vi "ST5520_CMD.vi"(8 "errin":errorcluster caption="entrée d'erreur (pas d'erreur)", 10 "VISA":string) -> (0 "errout":errorcluster caption="sortie d'erreur", 1 "DATA FINAL FLT":dbl, 2 "DATA OUT":string, 3 "60s?":bool)   [LabVIEW 2020]
uses:
  OP500/VG/VG_progressBar.vi
panel:
  in  "Arrêter":bool
  out "DATA LIVE":string
  # "DATA OUT"
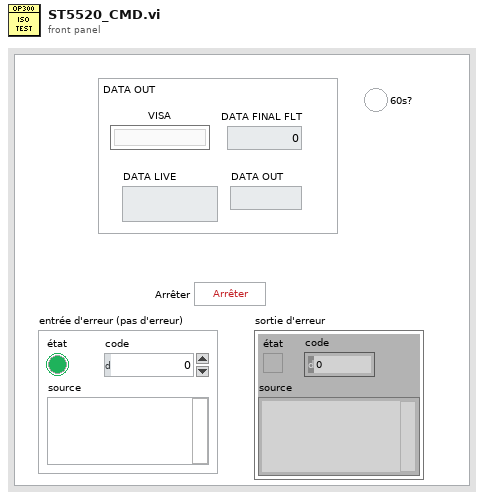
[diagram p1: front panel]
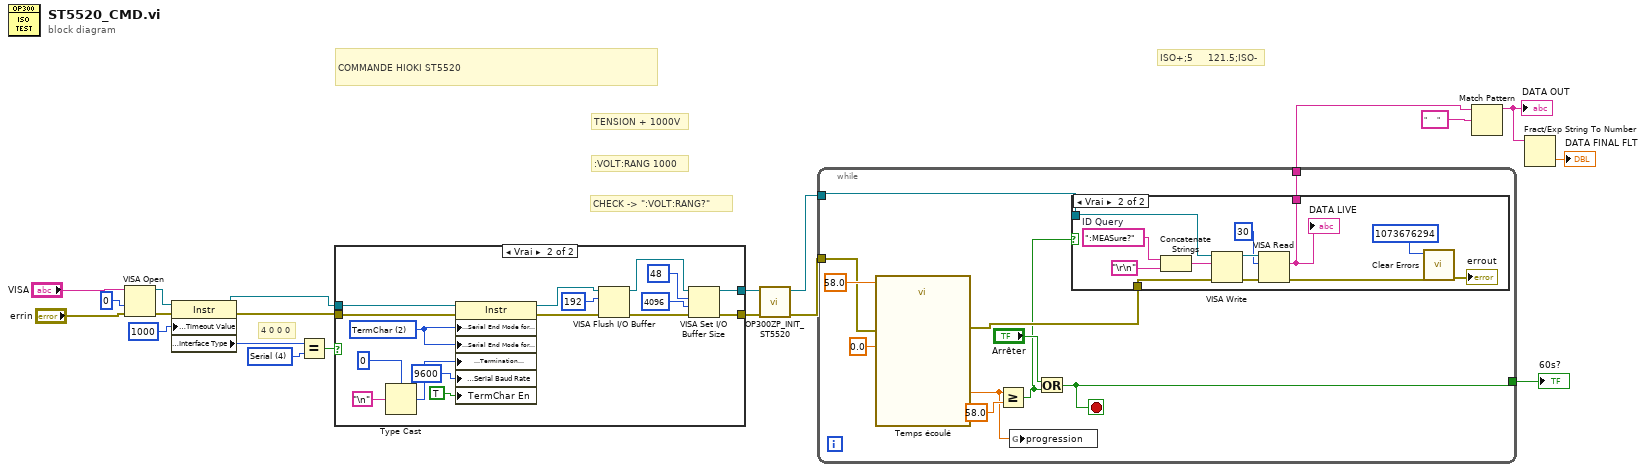
[diagram p0: block diagram]
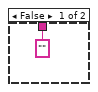
[diagram p3: hidden frame]
diagram:
  w11 = u16 4 items=["GPIB"=1, "VXI"=2, "GPIB-VXI"=3, "Serial"=4, "PXI"=5, "TCPIP"=6, "USB"=7] ("Interface Information:Interface Type")
  # "ISO+;5     121.5;ISO-"
  # "CHECK -> \":VOLT:RANG?\""
  # ":VOLT:RANG 1000"
  # "TENSION + 1000V"
  # "4 0 0 0"
  # "COMMANDE HIOKI ST5520"
  n1 = VISA Open(access mode=u32 0, error in (no error)="errin", VISA resource name="VISA") -> (VISA resource name=w13:refnum<visa-resource-name>, error out=w12:errorcluster)  [unwired: 2 in]
  n2 = property class="Instr"(reference=w13, error in=w12, "General Settings:Timeout Value"=u32 1000) -> (reference out=w8:refnum<visa-resource-name>, error out=w7:errorcluster, "Interface Information:Interface Type"=w10:u16)
  n3 = Equal?(x=w10, y=w11) -> (x = y?=w9:bool)
  n4 = case shown="Vrai" w9 {
    tunnel: [w21 w36] -> w5
    tunnel: [w22 w33] -> w6
    tunnel: w8 -> [w21 w38]
    tunnel: w7 -> [w22 w39]
    frame False {
      # "EDIT: Remove interfaces not supported by your instrument."
      # "GPIB, TCP/IP, and USB Interface"
    }
    frame True {
      w26 = u16 2 items=["None", "LastBit", "TermChar"] ("Serial Settings:Serial End Mode for Reads")
      n5 = Type Cast(type=u8 0, x="\n" ("Line Feed Constant")) -> (*(type *) &x=w25:u8)
      n6 = property class="Instr"(reference=w38, error in=w39, "Serial Settings:Serial End Mode for Reads"=w26, "Serial Settings:Serial End Mode for Writes"=w26, "Message Based Settings:Termination Character"=w25, "Serial Settings:Serial Baud Rate"=u32 9600 ("Serial Settings:Baud Rate"), "TermChar En"=TRUE ("Message Based Settings:Termination Character Enable")) -> (reference out=w32:refnum<visa-resource-name>, error out=w35:errorcluster)
      n7 = VISA Flush I/O Buffer(VISA resource name=w32, mask (16)=u16 192, error in (no error)=w35) -> (VISA resource name out=w37:refnum<visa-resource-name>, error out=w34:errorcluster)
      n8 = VISA Set I/O Buffer Size(VISA resource name=w37, mask (16)=u16 48, size (4096)=u32 4096 ("size (0)"), error in (no error)=w34) -> (VISA resource name out=w36:refnum<visa-resource-name>, error out=w33:errorcluster)
    }
  }
  n9 = call "OP300ZP_INIT_ST5520.vi"("errin"=w6, "VISA"=w5) -> ("errout"=w17:errorcluster, "VISA"=w18:refnum<visa-resource-name>)  [unwired: 8 in]
  n10 = while {
    tunnel: w17 -> [w44]
    tunnel: w18 -> [w50]
    tunnel: [w46] -> w2
    tunnel: [w45] -> w19
    stop <- w45 stop-if-true
    n11 = call "Temps écoulé"("Time Target (s)"=58.0, "error in (no error)"=w44, "Set Start Time (s)"=0.0) -> ("Elapsed Time (s)"=w41:dbl, "error out"=w42:errorcluster)  [unwired: 9 in, 6 out]
    n12 = Greater Or Equal?(x=w41, y=58.0) -> (x >= y?=w40:bool)
    n13 = global write "VG_progressBar.vi" "progression"(w41) -> ()
    n14 = Or(x="Arrêter", y=w40) -> (x .or. y?=w45:bool)
    n15 = case shown="Vrai" w40 {
      tunnel: w50 -> [_ w57]
      tunnel: ["" ("read buffer") w54] -> w46
      tunnel: w42 -> [_ w53]
      frame False {
      }
      frame True {
        w63 = ":MEASure?"  # ID Query
        n16 = Concatenate Strings(w63, "\r\n") -> (w59:string)
        n17 = VISA Write(VISA resource name=w57, write buffer=w59, error in (no error)=w53) -> (VISA resource name out=w62:refnum<visa-resource-name>, error out=w61:errorcluster)  [unwired: 1 out]
        n18 = VISA Read(VISA resource name=w62, byte count=u32 30 ("nombre d'octets"), error in (no error)=w61) -> (read buffer=w54:string, error out=w52:errorcluster)  [unwired: 2 out]
        "DATA LIVE" <- w54
        n19 = call <vilib>:"Clear Errors.vi"("error in (no error)"=w52, "specific error code to clear (0: all)"=1073676294) -> ("error out"=→"errout":errorcluster)  [unwired: 4 in, 1 out]
      }
    }
  }
  "60s?" <- w19
  n20 = Match Pattern(string=w2, regular expression="     " ("expression régulière")) -> (before substring=w1:string)  [unwired: 1 in, 3 out]
  "DATA OUT" <- w1
  n21 = Fract/Exp String To Number(string=w1) -> (number=→"DATA FINAL FLT":dbl)  [unwired: 3 in, 1 out]
